vi "Example- Detect IP In Bitfile.vi"() -> ()   [LabVIEW 2013]
uses:
  API/Engine Simulation IP.lvclass/Engine Simulation IP.ctl
  API/Engine Simulation Session.lvclass
  API/Engine Simulation IP.lvclass
  API/APU/APU.lvclass
  API/Analog Replay/Analog Replay.lvclass
  API/Digital Pattern Generation/Digital Pattern Generation.lvclass
panel:
  out "Digital Pattern Generation Names":string[](array[string])
  out "Analog Replay Names":string[](array[string])
  out "APU Names":string[](array[string])
  out "error out":errorcluster
  out "bitfile version":string
  in  "bitfile":path
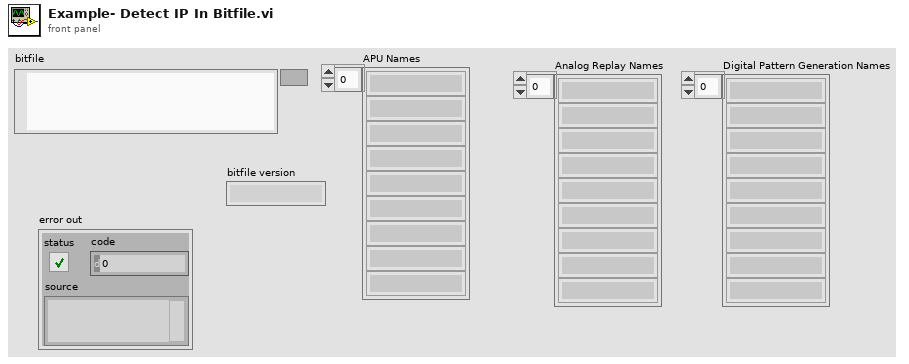
[diagram p1: front panel]
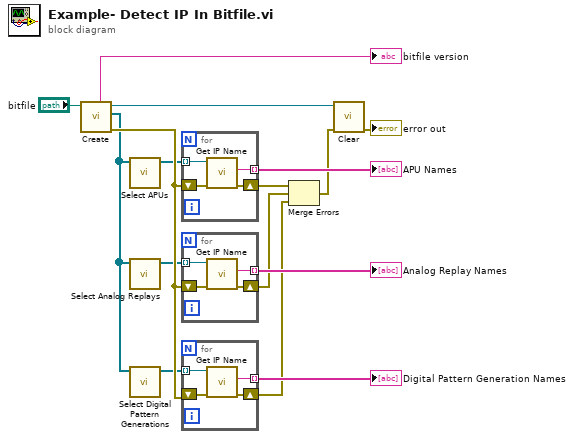
[diagram p0: block diagram]
diagram:
  n1 = call "Create.vi"("bitfile"="bitfile") -> ("error out"=w8:errorcluster, "IPs"=w4:refnum<class "Engine Simulation IP.lvclass">[], "Engine Simulation Session out"=w2:refnum<class "Engine Simulation Session.lvclass">, "bitfile full version"=→"bitfile version":string)  [unwired: 6 in, 1 out]
  n2 = call "Select APUs.vi"("IP"=w4) -> ("APUs"=w7:refnum<class "APU.lvclass">[])  [unwired: 10 in]
  n3 = call "Select Analog Replays.vi"("IP"=w4) -> ("analog replays"=w6:refnum<class "Analog Replay.lvclass">[])  [unwired: 10 in]
  n4 = call "Select Digital Pattern Generations.vi"("IP"=w4) -> ("digital patterns"=w5:refnum<class "Digital Pattern Generation.lvclass">[])  [unwired: 10 in]
  n5 = for {
    tunnel: w7 -> [w19] mode=indexing
    shift-right: [w18] -> w14
    shift-left: w8 -> [w20]
    tunnel: [w17] -> w15 mode=indexing
    n6 = call "Get IP Name.vi"("error in (no error)"=w20, "Engine Simulation IP in"=w19) -> ("error out"=w18:errorcluster, "Name"=w17:string)  [unwired: 7 in, 1 out]
  }
  "APU Names" <- w15
  n7 = for {
    tunnel: w6 -> [w23] mode=indexing
    shift-right: [w22] -> w10
    shift-left: w8 -> [w24]
    tunnel: [w21] -> w13 mode=indexing
    n8 = call "Get IP Name.vi"("error in (no error)"=w24, "Engine Simulation IP in"=w23) -> ("error out"=w22:errorcluster, "Name"=w21:string)  [unwired: 7 in, 1 out]
  }
  "Analog Replay Names" <- w13
  n9 = for {
    tunnel: w5 -> [w27] mode=indexing
    shift-right: [w26] -> w9
    shift-left: w8 -> [w28]
    tunnel: [w25] -> w12 mode=indexing
    n10 = call "Get IP Name.vi"("error in (no error)"=w28, "Engine Simulation IP in"=w27) -> ("error out"=w26:errorcluster, "Name"=w25:string)  [unwired: 7 in, 1 out]
  }
  "Digital Pattern Generation Names" <- w12
  n11 = Merge Errors(w14, w10, w9) -> (w3:errorcluster)
  n12 = call "Clear.vi"("error in (no error)"=w3, "Engine Simulation Session"=w2) -> ("error out"=→"error out":errorcluster)  [unwired: 9 in]
